vi "Voltage To Diode Close.vi"(8 "error in (no error)":errorcluster, 11 "Top Level in":refnum<class "Top Level.lvclass">) -> (0 "error out":errorcluster, 3 "Top Level out":refnum<class "Top Level.lvclass">)   [LabVIEW 2021, in "Top Level.lvlib" / "Top Level.lvclass"]
uses:
  Top Level.lvclass
  Top Level.lvclass/Top Level.ctl
  <vilib>/NathanCo/Analog Tasks/Analog Output/Analog Output/Analog Output.lvclass
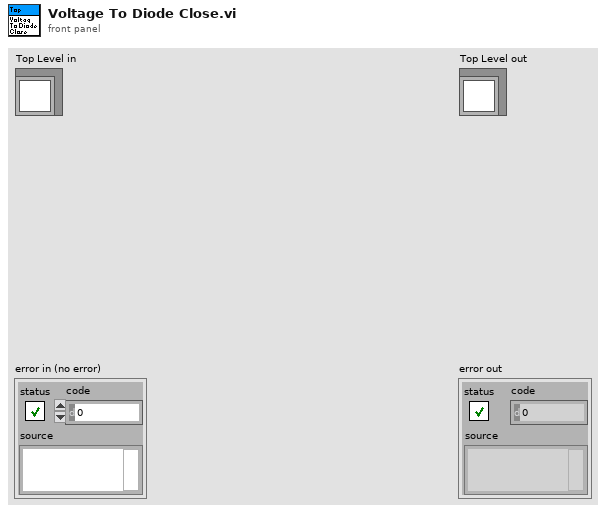
[diagram p1: front panel]
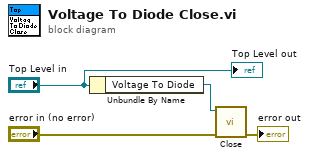
[diagram p0: block diagram]
diagram:
  n1 = Unbundle By Name("Top Level in") -> ("Voltage To Diode"=w4:refnum<class "Analog Output.lvclass">)
  n2 = call <vilib>:"Close.vi"("error in (no error)"="error in (no error)", "Analog Output in"=w4) -> ("error out"=→"error out":errorcluster)  [unwired: 9 in]
  "Top Level out" <- "Top Level in"
